vi "Create local tables from Server DB.vi"(6 "loadStatus Refnum":refnum<vi>, 8 "error in":errorcluster, 10 "Site":string="ICE1", 11 "tableNames":string[](array[string])) -> (0 "error out":errorcluster)   [LabVIEW 2015]
uses:
  <vilib>/addons/database/Auxilliary.llb/DB Tools DataTypes.ctl
  <vilib>/addons/database/Auxilliary.llb/DB Tools Cursor Type.ctl
  <vilib>/addons/database/Connection.llb/DB Tools Open Connec (Path).vi
  <vilib>/addons/database/Connection.llb/Conn Execute.vi
  <vilib>/addons/database/Recordset.llb/Rec Fetch Recordset Data (R).vi
  <vilib>/addons/database/Recordset.llb/Rec Destroy - Connection.vi
  <vilib>/addons/database/_DB Variant To Data/Database Variant To Data.xnode
  <vilib>/addons/database/NI_Database_API.lvlib
panel:
  out "column information":T2(array[cluster])
  out "columns":string[](array[string])
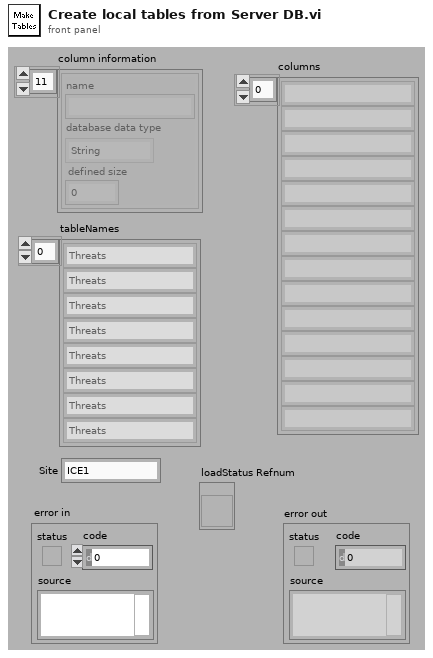
[diagram p1: front panel]
types:
  T1 = typedef "NI_Database_API.lvlib/DB Tools DataTypes.ctl" = enum16{"String", "Long (I32)", "Single (SGL)", "Double (DBL)", "Date/Time", "Binary"}
  T2 = cluster{"name":string, "database data type":T1, "defined size":i32}[]
  T3 = typedef "NI_Database_API.lvlib/DB Tools Cursor Type.ctl" = enum16{"forward-only", "keyset", "dynamic", "static"}
  T4 = typedef "NI_Database_API.lvlib/Conn ObjectReference.ctl" = refnum<k1>
  T5 = typedef "NI_Database_API.lvlib/Rec ObjectReference.ctl" = refnum<k1>
  T6 = cluster{"data":i32, "data":i32, "data":i32, "trimmed string":string, "trimmed string":string, "data":i32, "data":sgl, "data":i32, "data":i32, "data":i32, "trimmed string":string}
  T7 = cluster{"data":i32, "data":i32, "data":i32, "trimmed string":string, "data":i32, "data":i32, "trimmed string":string, "trimmed string":string, "trimmed string":string, "data":i32, "data":i32, "data":sgl, "data":i32, "data":i32, "trimmed string":string, "trimmed string":string}
  T8 = cluster{"data":i32, "trimmed string":string, "data":i32, "data":i32}
  T9 = cluster{"data":i32, "trimmed string":string, "data":i32, "trimmed string":string, "trimmed string":string, "trimmed string":string, "trimmed string":string, "data":sgl, "data":string, "trimmed string":string, "data":i32, "trimmed string":string, "trimmed string":string, "trimmed string":string}
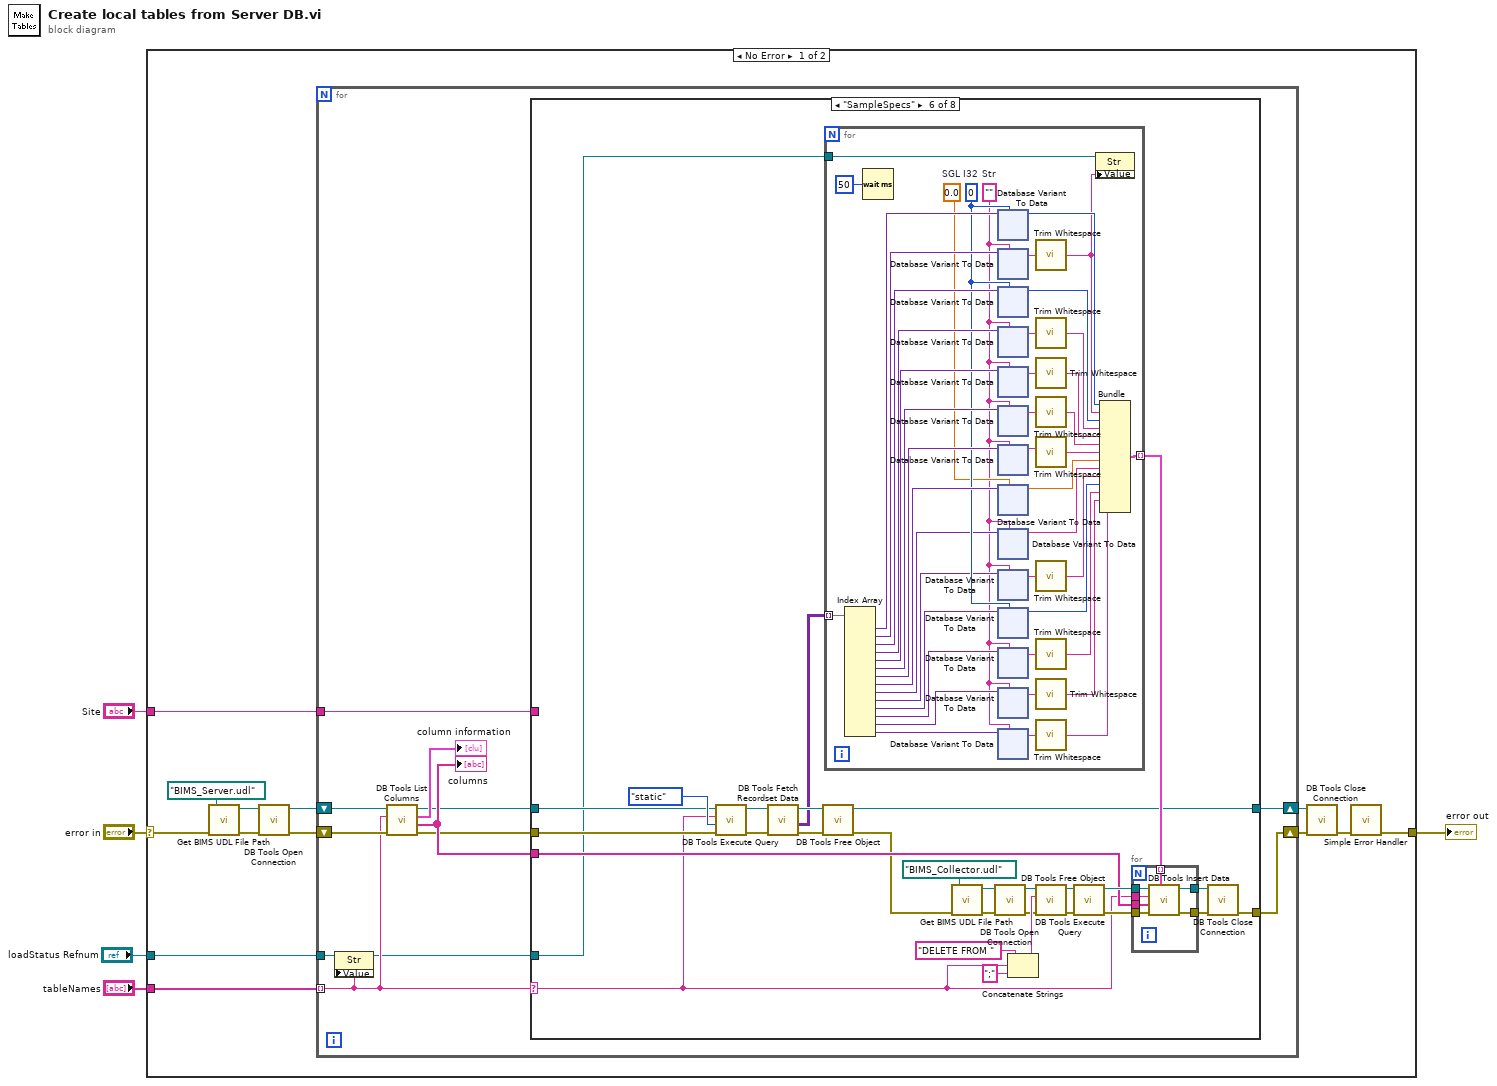
[diagram p0: block diagram]
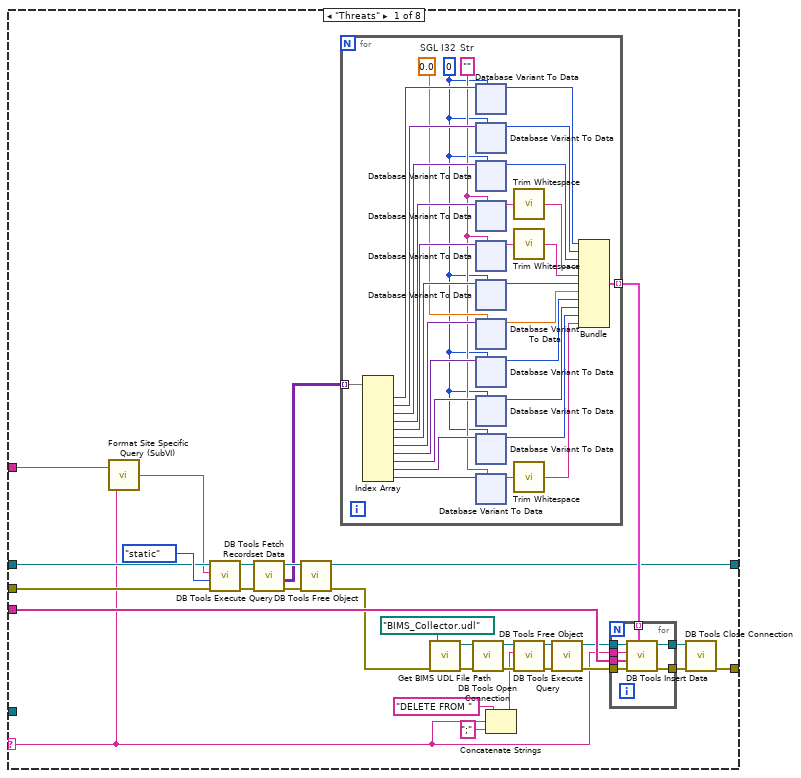
[diagram p2: hidden frame]
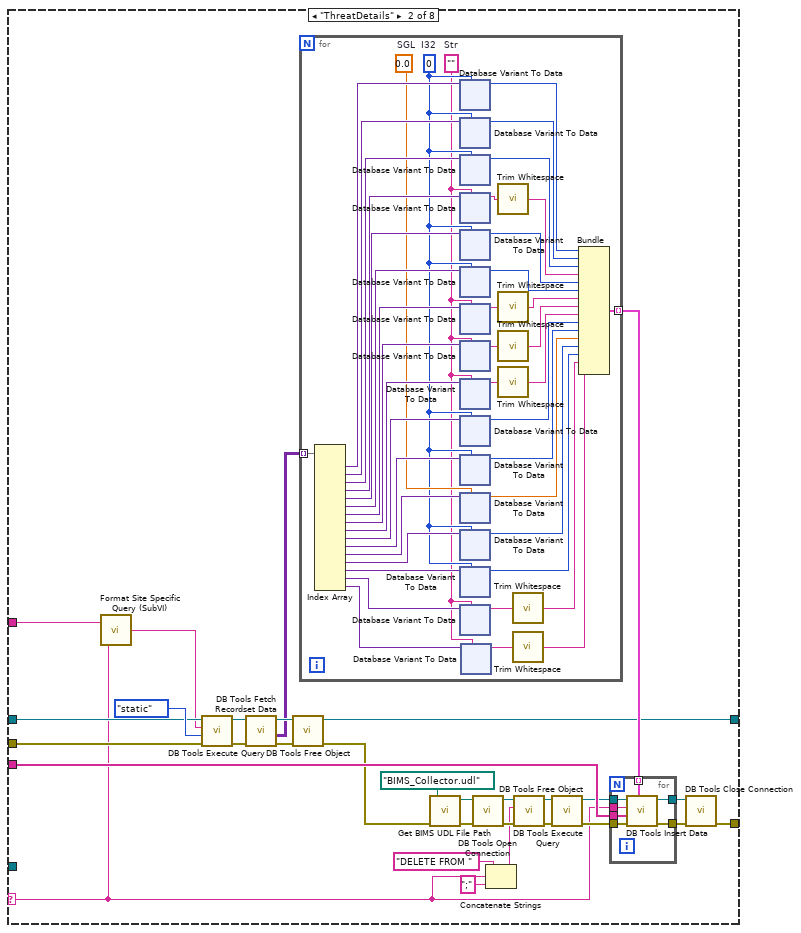
[diagram p3: hidden frame]
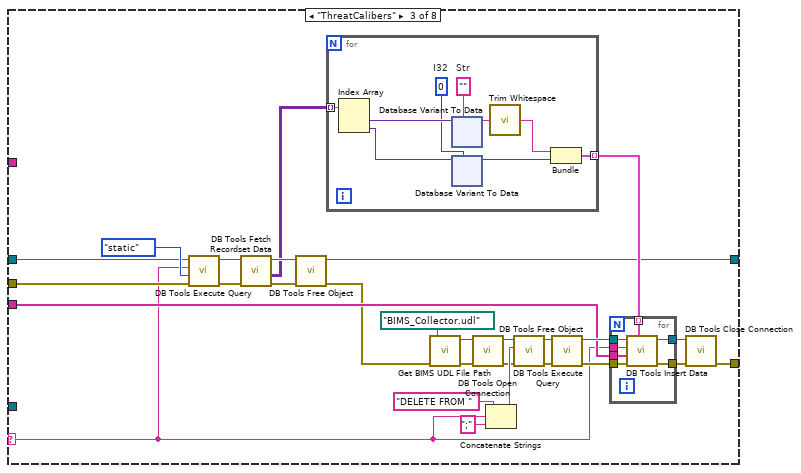
[diagram p4: hidden frame]
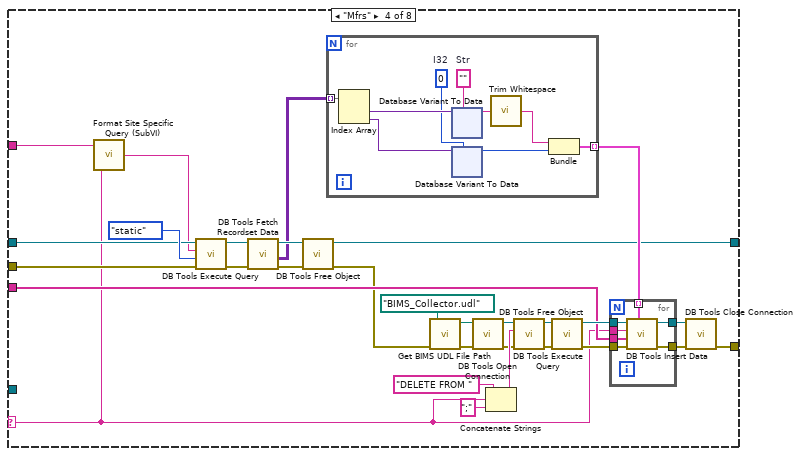
[diagram p5: hidden frame]
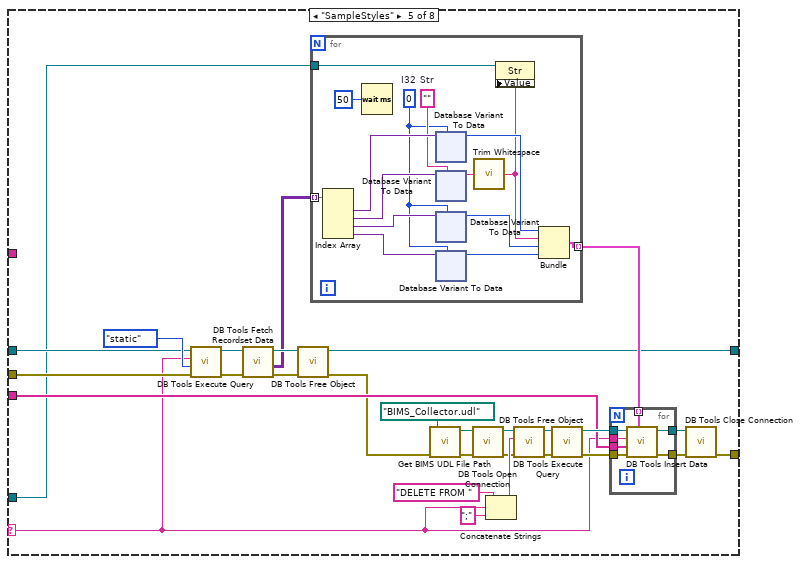
[diagram p6: hidden frame]
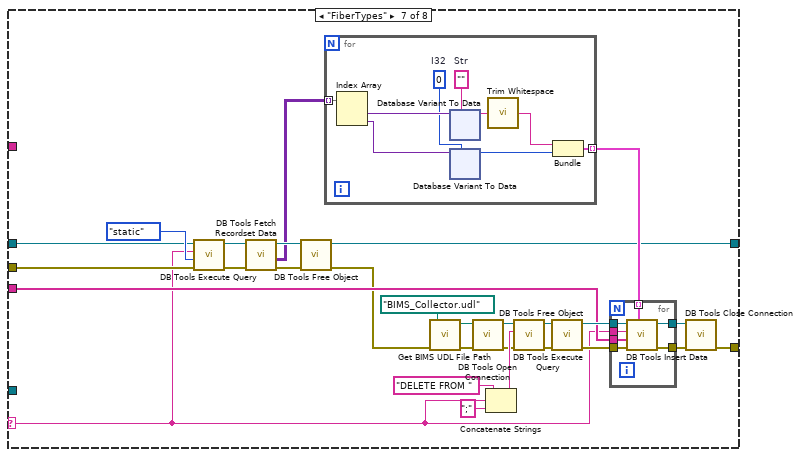
[diagram p7: hidden frame]
diagram:
  n1 = case shown="No Error" "error in" {
    selector: "error in" -> [w12 w2077]
    tunnel: [w16 w2077] -> w2
    tunnel: "tableNames" -> [w18 _]
    tunnel: "Site" -> [w17 _]
    tunnel: "loadStatus Refnum" -> [w6 _]
    frame No Error {
      n2 = call "Get BIMS UDL File Path.vi"("error in"=w12, "UDL file name"=path "BIMS_Server.udl") -> ("error out"=w15:errorcluster, "Full UDL file path"=w14:path)  [unwired: 4 out]
      n3 = call-poly <vilib>:"DB Tools Open Connection.vi"("error in (no error)"=w15, "connection information"=w14) -> ("error out"=w11:errorcluster, "connection reference"=w9:T4)  [unwired: 3 in, 3 out]
      n4 = for {
        tunnel: w18 -> [w20] mode=indexing
        shift-right: [w28] -> w8
        shift-left: w11 -> [w24]
        tunnel: w17 -> [w26]
        shift-right: [w23] -> w10
        shift-left: w9 -> [w22]
        tunnel: w6 -> [w21]
        n5 = property class="Str"(reference=w21, "Value"=w20) -> (reference out=w19:refnum<vi>)  [unwired: 1 in, 1 out]
        n6 = call <vilib>:"DB Tools List Columns.vi"("error in (no error)"=w24, "table"=w20, "connection reference"=w22) -> ("error out"=w27:errorcluster, "columns"=w29:string[], "column information"=→"column information":T2, "connection reference out"=w25:T4)  [unwired: 1 out]
        "columns" <- w29
        n7 = case shown="\"SampleSpecs\"" w20 {
          selector: w20 -> [w34 w453 w1046 w1154 w1265 w1440 w1971 _]
          tunnel: w27 -> [w39 w458 w1048 w1158 w1267 w1446 w1972 w2076]
          tunnel: w29 -> [w58 w477 w1055 w1165 w1274 w1454 w1981 _]
          tunnel: [w45 w464 w1054 w1164 w1273 w1453 w1980 w2076] -> w28
          tunnel: w25 -> [w38 w457 w1047 w1157 w1264 w1445 w1970 w2075]
          tunnel: w26 -> [w35 w454 _ w1155 _ _ _ _]
          tunnel: [w32 w450 w1043 w1151 w1262 w1442 w1967 w2075] -> w23
          tunnel: w19 -> [_ _ _ _ w1260 w1439 _ _]
          frame "Threats" {
            n8 = call "Format Site Specific Query (SubVI).vi"("Table"=w34, "Site"=w35) -> ("Query"=w36:string)
            n9 = call-poly <vilib>:"DB Tools Execute Query.vi"("error in (no error)"=w39, "cursor type"=DB_Tools_Cursor_Type."static", "SQL query"=w36, "connection reference"=w38) -> ("error out"=w43:errorcluster, "recordset reference"=w42:T5)  [unwired: 4 out]
            n10 = call-poly <vilib>:"DB Tools Fetch Recordset Data.vi"("error in (no error)"=w43, "recordset reference"=w42) -> ("error out"=w40:errorcluster, "recordset data"=w37:variant[][], "recordset reference out"=w41:T5)  [unwired: 3 out]
            n11 = call-poly <vilib>:"DB Tools Free Object.vi"("error in (no error)"=w40, "recordset reference"=w41) -> ("error out"=w31:errorcluster, "connection reference"=w32:T4)  [unwired: 8 out]
            n12 = for {
              tunnel: [w76] -> w55 mode=indexing
              tunnel: w37 -> [w97] mode=indexing
              w83 = sgl 0.0  # SGL
              w78 = ""  # Str
              w74 = 0  # I32
              n13 = Index Array(array=w97) -> (element #1=w96:variant, element #2=w95:variant, element #3=w92:variant, element #4=w91:variant, element #5=w90:variant, element #6=w89:variant, element #7=w88:variant, element #8=w87:variant, element #9=w82:variant, element #10=w80:variant, element #11=w77:variant)  [unwired: 11 in]
              n14 = xnode ("Database Variant To Data")("database variant"=w96, "type"=w74) -> ("data"=w75:i32)  [unwired: 1 in, 1 out]
              n15 = xnode "Database Variant To Data"("database variant"=w95, "type"=w74) -> ("data"=w94:i32)  [unwired: 1 in, 1 out]
              n16 = xnode "Database Variant To Data"("database variant"=w92, "type"=w74) -> ("data"=w93:i32)  [unwired: 1 in, 1 out]
              n17 = xnode "Database Variant To Data"("database variant"=w91, "type"=w78) -> ("data"=w73:string)  [unwired: 1 in, 1 out]
              n18 = xnode ("Database Variant To Data")("database variant"=w90, "type"=w78) -> ("data"=w71:string)  [unwired: 1 in, 1 out]
              n19 = xnode "Database Variant To Data"("database variant"=w89, "type"=w74) -> ("data"=w86:i32)  [unwired: 1 in, 1 out]
              n20 = xnode "Database Variant To Data"("database variant"=w88, "type"=w83) -> ("data"=w85:sgl)  [unwired: 1 in, 1 out]
              n21 = xnode "Database Variant To Data"("database variant"=w87, "type"=w74) -> ("data"=w84:i32)  [unwired: 1 in, 1 out]
              n22 = xnode "Database Variant To Data"("database variant"=w82, "type"=w74) -> ("data"=w81:i32)  [unwired: 1 in, 1 out]
              n23 = xnode "Database Variant To Data"("database variant"=w80, "type"=w74) -> ("data"=w79:i32)  [unwired: 1 in, 1 out]
              n24 = xnode "Database Variant To Data"("database variant"=w77, "type"=w78) -> ("data"=w69:string)  [unwired: 1 in, 1 out]
              n25 = call <vilib>:"Trim Whitespace.vi"("string"=w73) -> ("trimmed string"=w72:string)  [unwired: 1 in]
              n26 = call <vilib>:"Trim Whitespace.vi"("string"=w71) -> ("trimmed string"=w70:string)  [unwired: 1 in]
              n27 = call <vilib>:"Trim Whitespace.vi"("string"=w69) -> ("trimmed string"=w68:string)  [unwired: 1 in]
              n28 = Bundle("data"=w75, "data"=w94, "data"=w93, "trimmed string"=w72, "trimmed string"=w70, "data"=w86, "data"=w85, "data"=w84, "data"=w81, "data"=w79, "trimmed string"=w68) -> (w76:T6)  [unwired: 1 out]
            }
            n29 = call "Get BIMS UDL File Path.vi"("error in"=w31, "UDL file name"=path "BIMS_Collector.udl") -> ("error out"=w33:errorcluster, "Full UDL file path"=w60:path)  [unwired: 4 out]
            n30 = call-poly <vilib>:"DB Tools Open Connection.vi"("error in (no error)"=w33, "connection information"=w60) -> ("error out"=w54:errorcluster, "connection reference"=w51:T4)  [unwired: 3 in, 3 out]
            n31 = Concatenate Strings("DELETE FROM " ("SQL query"), w34, ";" ("string")) -> (w52:string)
            n32 = call-poly <vilib>:"DB Tools Execute Query.vi"("error in (no error)"=w54, "SQL query"=w52, "connection reference"=w51) -> ("error out"=w49:errorcluster, "recordset reference"=w47:T5)  [unwired: 1 in, 4 out]
            n33 = call-poly <vilib>:"DB Tools Free Object.vi"("error in (no error)"=w49, "recordset reference"=w47) -> ("error out"=w48:errorcluster, "connection reference"=w46:T4)  [unwired: 8 out]
            n34 = for {
              tunnel: [w67] -> w56
              tunnel: [w63] -> w57
              tunnel: w48 -> [w66]
              tunnel: w34 -> [w65]
              tunnel: w55 -> [w62] mode=indexing
              tunnel: w58 -> [w64]
              tunnel: w46 -> [w61]
              n35 = call <vilib>:"DB Tools Insert Data.vi"("data"=w62, "error in (no error)"=w66, "columns"=w64, "table"=w65, "connection reference"=w61) -> ("error out"=w63:errorcluster, "connection reference out"=w67:T4)  [unwired: 2 in, 3 out]
            }
            n36 = call <vilib>:"DB Tools Close Connection.vi"("error in (no error)"=w57, "connection reference"=w56) -> ("error out"=w45:errorcluster)  [unwired: 5 out]
          }
          frame "ThreatDetails" {
            n37 = call "Format Site Specific Query (SubVI).vi"("Table"=w453, "Site"=w454) -> ("Query"=w455:string)
            n38 = call-poly <vilib>:"DB Tools Execute Query.vi"("error in (no error)"=w458, "cursor type"=DB_Tools_Cursor_Type."static", "SQL query"=w455, "connection reference"=w457) -> ("error out"=w462:errorcluster, "recordset reference"=w461:T5)  [unwired: 4 out]
            n39 = call-poly <vilib>:"DB Tools Fetch Recordset Data.vi"("error in (no error)"=w462, "recordset reference"=w461) -> ("error out"=w459:errorcluster, "recordset data"=w456:variant[][], "recordset reference out"=w460:T5)  [unwired: 3 out]
            n40 = call-poly <vilib>:"DB Tools Free Object.vi"("error in (no error)"=w459, "recordset reference"=w460) -> ("error out"=w451:errorcluster, "connection reference"=w450:T4)  [unwired: 8 out]
            n41 = for {
              tunnel: [w513] -> w474 mode=indexing
              tunnel: w456 -> [w529] mode=indexing
              w500 = sgl 0.0  # SGL
              w489 = ""  # Str
              w496 = 0  # I32
              n42 = Index Array(array=w529) -> (element #1=w528:variant, element #2=w527:variant, element #3=w524:variant, element #4=w523:variant, element #5=w522:variant, element #6=w521:variant, element #7=w520:variant, element #8=w519:variant, element #9=w517:variant, element #10=w516:variant, element #11=w514:variant, element #12=w503:variant, element #13=w502:variant, element #14=w501:variant, element #15=w495:variant, element #16=w487:variant)  [unwired: 16 in]
              n43 = xnode ("Database Variant To Data")("database variant"=w528, "type"=w496) -> ("data"=w512:i32)  [unwired: 1 in, 1 out]
              n44 = xnode "Database Variant To Data"("database variant"=w527, "type"=w496) -> ("data"=w526:i32)  [unwired: 1 in, 1 out]
              n45 = xnode "Database Variant To Data"("database variant"=w524, "type"=w496) -> ("data"=w525:i32)  [unwired: 1 in, 1 out]
              n46 = xnode "Database Variant To Data"("database variant"=w523, "type"=w489) -> ("data"=w511:string)  [unwired: 1 in, 1 out]
              n47 = xnode ("Database Variant To Data")("database variant"=w522, "type"=w496) -> ("data"=w509:i32)  [unwired: 1 in, 1 out]
              n48 = xnode "Database Variant To Data"("database variant"=w521, "type"=w496) -> ("data"=w518:i32)  [unwired: 1 in, 1 out]
              n49 = xnode "Database Variant To Data"("database variant"=w520, "type"=w489) -> ("data"=w492:string)  [unwired: 1 in, 1 out]
              n50 = xnode "Database Variant To Data"("database variant"=w519, "type"=w489) -> ("data"=w508:string)  [unwired: 1 in, 1 out]
              n51 = xnode "Database Variant To Data"("database variant"=w517, "type"=w489) -> ("data"=w506:string)  [unwired: 1 in, 1 out]
              n52 = xnode "Database Variant To Data"("database variant"=w516, "type"=w496) -> ("data"=w515:i32)  [unwired: 1 in, 1 out]
              n53 = xnode "Database Variant To Data"("database variant"=w514, "type"=w496) -> ("data"=w504:i32)  [unwired: 1 in, 1 out]
              n54 = xnode "Database Variant To Data"("database variant"=w503, "type"=w500) -> ("data"=w499:sgl)  [unwired: 1 in, 1 out]
              n55 = xnode "Database Variant To Data"("database variant"=w502, "type"=w496) -> ("data"=w498:i32)  [unwired: 1 in, 1 out]
              n56 = xnode "Database Variant To Data"("database variant"=w501, "type"=w496) -> ("data"=w497:i32)  [unwired: 1 in, 1 out]
              n57 = xnode "Database Variant To Data"("database variant"=w495, "type"=w489) -> ("data"=w494:string)  [unwired: 1 in, 1 out]
              n58 = xnode "Database Variant To Data"("database variant"=w487, "type"=w489) -> ("data"=w490:string)  [unwired: 1 in, 1 out]
              n59 = call <vilib>:"Trim Whitespace.vi"("string"=w511) -> ("trimmed string"=w510:string)  [unwired: 1 in]
              n60 = call <vilib>:"Trim Whitespace.vi"("string"=w492) -> ("trimmed string"=w491:string)  [unwired: 1 in]
              n61 = call <vilib>:"Trim Whitespace.vi"("string"=w508) -> ("trimmed string"=w507:string)  [unwired: 1 in]
              n62 = call <vilib>:"Trim Whitespace.vi"("string"=w506) -> ("trimmed string"=w505:string)  [unwired: 1 in]
              n63 = call <vilib>:"Trim Whitespace.vi"("string"=w494) -> ("trimmed string"=w493:string)  [unwired: 1 in]
              n64 = call <vilib>:"Trim Whitespace.vi"("string"=w490) -> ("trimmed string"=w488:string)  [unwired: 1 in]
              n65 = Bundle("data"=w512, "data"=w526, "data"=w525, "trimmed string"=w510, "data"=w509, "data"=w518, "trimmed string"=w491, "trimmed string"=w507, "trimmed string"=w505, "data"=w515, "data"=w504, "data"=w499, "data"=w498, "data"=w497, "trimmed string"=w493, "trimmed string"=w488) -> (w513:T7)  [unwired: 1 out]
            }
            n66 = call "Get BIMS UDL File Path.vi"("error in"=w451, "UDL file name"=path "BIMS_Collector.udl") -> ("error out"=w452:errorcluster, "Full UDL file path"=w479:path)  [unwired: 4 out]
            n67 = call-poly <vilib>:"DB Tools Open Connection.vi"("error in (no error)"=w452, "connection information"=w479) -> ("error out"=w473:errorcluster, "connection reference"=w470:T4)  [unwired: 3 in, 3 out]
            n68 = Concatenate Strings("DELETE FROM " ("SQL query"), w453, ";" ("string")) -> (w471:string)
            n69 = call-poly <vilib>:"DB Tools Execute Query.vi"("error in (no error)"=w473, "SQL query"=w471, "connection reference"=w470) -> ("error out"=w468:errorcluster, "recordset reference"=w466:T5)  [unwired: 1 in, 4 out]
            n70 = call-poly <vilib>:"DB Tools Free Object.vi"("error in (no error)"=w468, "recordset reference"=w466) -> ("error out"=w467:errorcluster, "connection reference"=w465:T4)  [unwired: 8 out]
            n71 = for {
              tunnel: [w486] -> w475
              tunnel: [w482] -> w476
              tunnel: w467 -> [w485]
              tunnel: w453 -> [w484]
              tunnel: w474 -> [w481] mode=indexing
              tunnel: w477 -> [w483]
              tunnel: w465 -> [w480]
              n72 = call <vilib>:"DB Tools Insert Data.vi"("data"=w481, "error in (no error)"=w485, "columns"=w483, "table"=w484, "connection reference"=w480) -> ("error out"=w482:errorcluster, "connection reference out"=w486:T4)  [unwired: 2 in, 3 out]
            }
            n73 = call <vilib>:"DB Tools Close Connection.vi"("error in (no error)"=w476, "connection reference"=w475) -> ("error out"=w464:errorcluster)  [unwired: 5 out]
          }
          frame "ThreatCalibers" {
            n74 = call-poly <vilib>:"DB Tools Execute Query.vi"("error in (no error)"=w1048, "cursor type"=DB_Tools_Cursor_Type."static", "SQL query"=w1046, "connection reference"=w1047) -> ("error out"=w1051:errorcluster, "recordset reference"=w1050:T5)  [unwired: 4 out]
            n75 = call-poly <vilib>:"DB Tools Fetch Recordset Data.vi"("error in (no error)"=w1051, "recordset reference"=w1050) -> ("error out"=w1052:errorcluster, "recordset data"=w1045:variant[][], "recordset reference out"=w1049:T5)  [unwired: 3 out]
            n76 = call-poly <vilib>:"DB Tools Free Object.vi"("error in (no error)"=w1052, "recordset reference"=w1049) -> ("error out"=w1042:errorcluster, "connection reference"=w1043:T4)  [unwired: 8 out]
            n77 = for {
              tunnel: [w1081] -> w1060 mode=indexing
              tunnel: w1045 -> [w1085] mode=indexing
              w1077 = ""  # Str
              w1078 = 0  # I32
              n78 = Index Array(array=w1085) -> (element #1=w1084:variant, element #2=w1083:variant)  [unwired: 2 in]
              n79 = xnode ("Database Variant To Data")("database variant"=w1084, "type"=w1077) -> ("data"=w1080:string)  [unwired: 1 in, 1 out]
              n80 = xnode "Database Variant To Data"("database variant"=w1083, "type"=w1078) -> ("data"=w1082:i32)  [unwired: 1 in, 1 out]
              n81 = call <vilib>:"Trim Whitespace.vi"("string"=w1080) -> ("trimmed string"=w1079:string)  [unwired: 1 in]
              n82 = Bundle("trimmed string"=w1079, "data"=w1082) -> (w1081:cluster{"trimmed string":string, "data":i32})  [unwired: 1 out]
            }
            n83 = call "Get BIMS UDL File Path.vi"("error in"=w1042, "UDL file name"=path "BIMS_Collector.udl") -> ("error out"=w1044:errorcluster, "Full UDL file path"=w1056:path)  [unwired: 4 out]
            n84 = call-poly <vilib>:"DB Tools Open Connection.vi"("error in (no error)"=w1044, "connection information"=w1056) -> ("error out"=w1061:errorcluster, "connection reference"=w1064:T4)  [unwired: 3 in, 3 out]
            n85 = Concatenate Strings("DELETE FROM " ("SQL query"), w1046, ";" ("string")) -> (w1063:string)
            n86 = call-poly <vilib>:"DB Tools Execute Query.vi"("error in (no error)"=w1061, "SQL query"=w1063, "connection reference"=w1064) -> ("error out"=w1066:errorcluster, "recordset reference"=w1068:T5)  [unwired: 1 in, 4 out]
            n87 = call-poly <vilib>:"DB Tools Free Object.vi"("error in (no error)"=w1066, "recordset reference"=w1068) -> ("error out"=w1067:errorcluster, "connection reference"=w1069:T4)  [unwired: 8 out]
            n88 = for {
              tunnel: [w1076] -> w1059
              tunnel: [w1072] -> w1058
              tunnel: w1067 -> [w1075]
              tunnel: w1046 -> [w1074]
              tunnel: w1060 -> [w1071] mode=indexing
              tunnel: w1055 -> [w1073]
              tunnel: w1069 -> [w1070]
              n89 = call <vilib>:"DB Tools Insert Data.vi"("data"=w1071, "error in (no error)"=w1075, "columns"=w1073, "table"=w1074, "connection reference"=w1070) -> ("error out"=w1072:errorcluster, "connection reference out"=w1076:T4)  [unwired: 2 in, 3 out]
            }
            n90 = call <vilib>:"DB Tools Close Connection.vi"("error in (no error)"=w1058, "connection reference"=w1059) -> ("error out"=w1054:errorcluster)  [unwired: 5 out]
          }
          frame "Mfrs" {
            n91 = call "Format Site Specific Query (SubVI).vi"("Table"=w1154, "Site"=w1155) -> ("Query"=w1153:string)
            n92 = call-poly <vilib>:"DB Tools Execute Query.vi"("error in (no error)"=w1158, "cursor type"=DB_Tools_Cursor_Type."static", "SQL query"=w1153, "connection reference"=w1157) -> ("error out"=w1161:errorcluster, "recordset reference"=w1160:T5)  [unwired: 4 out]
            n93 = call-poly <vilib>:"DB Tools Fetch Recordset Data.vi"("error in (no error)"=w1161, "recordset reference"=w1160) -> ("error out"=w1162:errorcluster, "recordset data"=w1156:variant[][], "recordset reference out"=w1159:T5)  [unwired: 3 out]
            n94 = call-poly <vilib>:"DB Tools Free Object.vi"("error in (no error)"=w1162, "recordset reference"=w1159) -> ("error out"=w1150:errorcluster, "connection reference"=w1151:T4)  [unwired: 8 out]
            n95 = for {
              tunnel: [w1193] -> w1170 mode=indexing
              tunnel: w1156 -> [w1195] mode=indexing
              w1190 = ""  # Str
              w1189 = 0  # I32
              n96 = Index Array(array=w1195) -> (element #1=w1191:variant, element #2=w1194:variant)  [unwired: 2 in]
              n97 = xnode "Database Variant To Data"("database variant"=w1191, "type"=w1190) -> ("data"=w1188:string)  [unwired: 1 in, 1 out]
              n98 = xnode ("Database Variant To Data")("database variant"=w1194, "type"=w1189) -> ("data"=w1187:i32)  [unwired: 1 in, 1 out]
              n99 = call <vilib>:"Trim Whitespace.vi"("string"=w1188) -> ("trimmed string"=w1192:string)  [unwired: 1 in]
              n100 = Bundle("trimmed string"=w1192, "data"=w1187) -> (w1193:cluster{"trimmed string":string, "data":i32})  [unwired: 1 out]
            }
            n101 = call "Get BIMS UDL File Path.vi"("error in"=w1150, "UDL file name"=path "BIMS_Collector.udl") -> ("error out"=w1152:errorcluster, "Full UDL file path"=w1166:path)  [unwired: 4 out]
            n102 = call-poly <vilib>:"DB Tools Open Connection.vi"("error in (no error)"=w1152, "connection information"=w1166) -> ("error out"=w1171:errorcluster, "connection reference"=w1174:T4)  [unwired: 3 in, 3 out]
            n103 = Concatenate Strings("DELETE FROM " ("SQL query"), w1154, ";" ("string")) -> (w1173:string)
            n104 = call-poly <vilib>:"DB Tools Execute Query.vi"("error in (no error)"=w1171, "SQL query"=w1173, "connection reference"=w1174) -> ("error out"=w1176:errorcluster, "recordset reference"=w1178:T5)  [unwired: 1 in, 4 out]
            n105 = call-poly <vilib>:"DB Tools Free Object.vi"("error in (no error)"=w1176, "recordset reference"=w1178) -> ("error out"=w1177:errorcluster, "connection reference"=w1179:T4)  [unwired: 8 out]
            n106 = for {
              tunnel: [w1186] -> w1169
              tunnel: [w1182] -> w1168
              tunnel: w1177 -> [w1185]
              tunnel: w1154 -> [w1184]
              tunnel: w1170 -> [w1181] mode=indexing
              tunnel: w1165 -> [w1183]
              tunnel: w1179 -> [w1180]
              n107 = call <vilib>:"DB Tools Insert Data.vi"("data"=w1181, "error in (no error)"=w1185, "columns"=w1183, "table"=w1184, "connection reference"=w1180) -> ("error out"=w1182:errorcluster, "connection reference out"=w1186:T4)  [unwired: 2 in, 3 out]
            }
            n108 = call <vilib>:"DB Tools Close Connection.vi"("error in (no error)"=w1168, "connection reference"=w1169) -> ("error out"=w1164:errorcluster)  [unwired: 5 out]
          }
          frame "SampleStyles" {
            n109 = call-poly <vilib>:"DB Tools Execute Query.vi"("error in (no error)"=w1267, "cursor type"=DB_Tools_Cursor_Type."static", "SQL query"=w1265, "connection reference"=w1264) -> ("error out"=w1270:errorcluster, "recordset reference"=w1269:T5)  [unwired: 4 out]
            n110 = call-poly <vilib>:"DB Tools Fetch Recordset Data.vi"("error in (no error)"=w1270, "recordset reference"=w1269) -> ("error out"=w1271:errorcluster, "recordset data"=w1266:variant[][], "recordset reference out"=w1268:T5)  [unwired: 3 out]
            n111 = call-poly <vilib>:"DB Tools Free Object.vi"("error in (no error)"=w1271, "recordset reference"=w1268) -> ("error out"=w1261:errorcluster, "connection reference"=w1262:T4)  [unwired: 8 out]
            n112 = for {
              tunnel: [w1306] -> w1279 mode=indexing
              tunnel: w1266 -> [w1310] mode=indexing
              tunnel: w1260 -> [w1298]
              w1303 = ""  # Str
              w1302 = 0  # I32
              n113 = Index Array(array=w1310) -> (element #1=w1304:variant, element #2=w1305:variant, element #3=w1309:variant, element #4=w1308:variant)  [unwired: 4 in]
              n114 = Wait (ms)(milliseconds to wait=u32 50) -> ()  [unwired: 1 out]
              n115 = xnode ("Database Variant To Data")("database variant"=w1304, "type"=w1302) -> ("data"=w1300:i32)  [unwired: 1 in, 1 out]
              n116 = xnode "Database Variant To Data"("database variant"=w1305, "type"=w1303) -> ("data"=w1301:string)  [unwired: 1 in, 1 out]
              n117 = xnode ("Database Variant To Data")("database variant"=w1309, "type"=w1302) -> ("data"=w1299:i32)  [unwired: 1 in, 1 out]
              n118 = xnode "Database Variant To Data"("database variant"=w1308, "type"=w1302) -> ("data"=w1307:i32)  [unwired: 1 in, 1 out]
              n119 = call <vilib>:"Trim Whitespace.vi"("string"=w1301) -> ("trimmed string"=w1297:string)  [unwired: 1 in]
              n120 = property class="Str"(reference=w1298, "Value"=w1297) -> ()  [unwired: 1 in, 2 out]
              n121 = Bundle("data"=w1300, "trimmed string"=w1297, "data"=w1299, "data"=w1307) -> (w1306:T8)  [unwired: 1 out]
            }
            n122 = call "Get BIMS UDL File Path.vi"("error in"=w1261, "UDL file name"=path "BIMS_Collector.udl") -> ("error out"=w1263:errorcluster, "Full UDL file path"=w1275:path)  [unwired: 4 out]
            n123 = call-poly <vilib>:"DB Tools Open Connection.vi"("error in (no error)"=w1263, "connection information"=w1275) -> ("error out"=w1280:errorcluster, "connection reference"=w1283:T4)  [unwired: 3 in, 3 out]
            n124 = Concatenate Strings("DELETE FROM " ("SQL query"), w1265, ";" ("string")) -> (w1282:string)
            n125 = call-poly <vilib>:"DB Tools Execute Query.vi"("error in (no error)"=w1280, "SQL query"=w1282, "connection reference"=w1283) -> ("error out"=w1285:errorcluster, "recordset reference"=w1287:T5)  [unwired: 1 in, 4 out]
            n126 = call-poly <vilib>:"DB Tools Free Object.vi"("error in (no error)"=w1285, "recordset reference"=w1287) -> ("error out"=w1286:errorcluster, "connection reference"=w1288:T4)  [unwired: 8 out]
            n127 = for {
              tunnel: [w1295] -> w1278
              tunnel: [w1291] -> w1277
              tunnel: w1286 -> [w1294]
              tunnel: w1265 -> [w1293]
              tunnel: w1279 -> [w1290] mode=indexing
              tunnel: w1274 -> [w1292]
              tunnel: w1288 -> [w1289]
              n128 = call <vilib>:"DB Tools Insert Data.vi"("data"=w1290, "error in (no error)"=w1294, "columns"=w1292, "table"=w1293, "connection reference"=w1289) -> ("error out"=w1291:errorcluster, "connection reference out"=w1295:T4)  [unwired: 2 in, 3 out]
            }
            n129 = call <vilib>:"DB Tools Close Connection.vi"("error in (no error)"=w1277, "connection reference"=w1278) -> ("error out"=w1273:errorcluster)  [unwired: 5 out]
          }
          frame "SampleSpecs" {
            n130 = call-poly <vilib>:"DB Tools Execute Query.vi"("error in (no error)"=w1446, "cursor type"=DB_Tools_Cursor_Type."static", "SQL query"=w1440, "connection reference"=w1445) -> ("error out"=w1449:errorcluster, "recordset reference"=w1448:T5)  [unwired: 4 out]
            n131 = call-poly <vilib>:"DB Tools Fetch Recordset Data.vi"("error in (no error)"=w1449, "recordset reference"=w1448) -> ("error out"=w1450:errorcluster, "recordset data"=w1444:variant[][], "recordset reference out"=w1447:T5)  [unwired: 3 out]
            n132 = call-poly <vilib>:"DB Tools Free Object.vi"("error in (no error)"=w1450, "recordset reference"=w1447) -> ("error out"=w1441:errorcluster, "connection reference"=w1442:T4)  [unwired: 8 out]
            n133 = for {
              tunnel: [w1499] -> w1452 mode=indexing
              tunnel: w1444 -> [w1511] mode=indexing
              tunnel: w1439 -> [w1468]
              w1475 = sgl 0.0  # SGL
              w1472 = ""  # Str
              w1497 = 0  # I32
              n134 = Index Array(array=w1511) -> (element #1=w1510:variant, element #2=w1509:variant, element #3=w1507:variant, element #4=w1506:variant, element #5=w1505:variant, element #6=w1504:variant, element #7=w1503:variant, element #8=w1502:variant, element #9=w1476:variant, element #10=w1477:variant, element #11=w1478:variant, element #12=w1479:variant, element #13=w1480:variant, element #14=w1473:variant)  [unwired: 14 in]
              n135 = Wait (ms)(milliseconds to wait=u32 50) -> ()  [unwired: 1 out]
              n136 = xnode ("Database Variant To Data")("database variant"=w1510, "type"=w1497) -> ("data"=w1498:i32)  [unwired: 1 in, 1 out]
              n137 = xnode "Database Variant To Data"("database variant"=w1509, "type"=w1472) -> ("data"=w1490:string)  [unwired: 1 in, 1 out]
              n138 = xnode "Database Variant To Data"("database variant"=w1507, "type"=w1497) -> ("data"=w1508:i32)  [unwired: 1 in, 1 out]
              n139 = xnode "Database Variant To Data"("database variant"=w1506, "type"=w1472) -> ("data"=w1496:string)  [unwired: 1 in, 1 out]
              n140 = xnode ("Database Variant To Data")("database variant"=w1505, "type"=w1472) -> ("data"=w1494:string)  [unwired: 1 in, 1 out]
              n141 = xnode "Database Variant To Data"("database variant"=w1504, "type"=w1472) -> ("data"=w1485:string)  [unwired: 1 in, 1 out]
              n142 = xnode "Database Variant To Data"("database variant"=w1503, "type"=w1472) -> ("data"=w1487:string)  [unwired: 1 in, 1 out]
              n143 = xnode "Database Variant To Data"("database variant"=w1502, "type"=w1475) -> ("data"=w1501:sgl)  [unwired: 1 in, 1 out]
              n144 = xnode "Database Variant To Data"("database variant"=w1476, "type"=w1472) -> ("data"=w1481:string)  [unwired: 1 in, 1 out]
              n145 = xnode "Database Variant To Data"("database variant"=w1477, "type"=w1472) -> ("data"=w1489:string)  [unwired: 1 in, 1 out]
              n146 = xnode "Database Variant To Data"("database variant"=w1478, "type"=w1497) -> ("data"=w1500:i32)  [unwired: 1 in, 1 out]
              n147 = xnode "Database Variant To Data"("database variant"=w1479, "type"=w1472) -> ("data"=w1492:string)  [unwired: 1 in, 1 out]
              n148 = xnode "Database Variant To Data"("database variant"=w1480, "type"=w1472) -> ("data"=w1483:string)  [unwired: 1 in, 1 out]
              n149 = xnode "Database Variant To Data"("database variant"=w1473, "type"=w1472) -> ("data"=w1474:string)  [unwired: 1 in, 1 out]
              n150 = call <vilib>:"Trim Whitespace.vi"("string"=w1490) -> ("trimmed string"=w1469:string)  [unwired: 1 in]
              n151 = call <vilib>:"Trim Whitespace.vi"("string"=w1496) -> ("trimmed string"=w1495:string)  [unwired: 1 in]
              n152 = call <vilib>:"Trim Whitespace.vi"("string"=w1494) -> ("trimmed string"=w1493:string)  [unwired: 1 in]
              n153 = call <vilib>:"Trim Whitespace.vi"("string"=w1485) -> ("trimmed string"=w1484:string)  [unwired: 1 in]
              n154 = call <vilib>:"Trim Whitespace.vi"("string"=w1487) -> ("trimmed string"=w1486:string)  [unwired: 1 in]
              n155 = call <vilib>:"Trim Whitespace.vi"("string"=w1489) -> ("trimmed string"=w1488:string)  [unwired: 1 in]
              n156 = call <vilib>:"Trim Whitespace.vi"("string"=w1492) -> ("trimmed string"=w1491:string)  [unwired: 1 in]
              n157 = call <vilib>:"Trim Whitespace.vi"("string"=w1483) -> ("trimmed string"=w1482:string)  [unwired: 1 in]
              n158 = call <vilib>:"Trim Whitespace.vi"("string"=w1474) -> ("trimmed string"=w1471:string)  [unwired: 1 in]
              n159 = property class="Str"(reference=w1468, "Value"=w1469) -> ()  [unwired: 1 in, 2 out]
              n160 = Bundle("data"=w1498, "trimmed string"=w1469, "data"=w1508, "trimmed string"=w1495, "trimmed string"=w1493, "trimmed string"=w1484, "trimmed string"=w1486, "data"=w1501, "data"=w1481, "trimmed string"=w1488, "data"=w1500, "trimmed string"=w1491, "trimmed string"=w1482, "trimmed string"=w1471) -> (w1499:T9)  [unwired: 1 out]
            }
            n161 = call "Get BIMS UDL File Path.vi"("error in"=w1441, "UDL file name"=path "BIMS_Collector.udl") -> ("error out"=w1443:errorcluster, "Full UDL file path"=w1455:path)  [unwired: 4 out]
            n162 = call-poly <vilib>:"DB Tools Open Connection.vi"("error in (no error)"=w1443, "connection information"=w1455) -> ("error out"=w1459:errorcluster, "connection reference"=w1462:T4)  [unwired: 3 in, 3 out]
            n163 = Concatenate Strings("DELETE FROM " ("SQL query"), w1440, ";" ("string")) -> (w1461:string)
            n164 = call-poly <vilib>:"DB Tools Execute Query.vi"("error in (no error)"=w1459, "SQL query"=w1461, "connection reference"=w1462) -> ("error out"=w1464:errorcluster, "recordset reference"=w1466:T5)  [unwired: 1 in, 4 out]
            n165 = call-poly <vilib>:"DB Tools Free Object.vi"("error in (no error)"=w1464, "recordset reference"=w1466) -> ("error out"=w1465:errorcluster, "connection reference"=w1467:T4)  [unwired: 8 out]
            n166 = for {
              tunnel: [w1966] -> w1458
              tunnel: [w1962] -> w1457
              tunnel: w1465 -> [w1965]
              tunnel: w1440 -> [w1964]
              tunnel: w1452 -> [w1961] mode=indexing
              tunnel: w1454 -> [w1963]
              tunnel: w1467 -> [w1960]
              n167 = call <vilib>:"DB Tools Insert Data.vi"("data"=w1961, "error in (no error)"=w1965, "columns"=w1963, "table"=w1964, "connection reference"=w1960) -> ("error out"=w1962:errorcluster, "connection reference out"=w1966:T4)  [unwired: 2 in, 3 out]
            }
            n168 = call <vilib>:"DB Tools Close Connection.vi"("error in (no error)"=w1457, "connection reference"=w1458) -> ("error out"=w1453:errorcluster)  [unwired: 5 out]
          }
          frame "FiberTypes" {
            n169 = call-poly <vilib>:"DB Tools Execute Query.vi"("error in (no error)"=w1972, "cursor type"=DB_Tools_Cursor_Type."static", "SQL query"=w1971, "connection reference"=w1970) -> ("error out"=w1977:errorcluster, "recordset reference"=w1976:T5)  [unwired: 4 out]
            n170 = call-poly <vilib>:"DB Tools Fetch Recordset Data.vi"("error in (no error)"=w1977, "recordset reference"=w1976) -> ("error out"=w1974:errorcluster, "recordset data"=w1973:variant[][], "recordset reference out"=w1975:T5)  [unwired: 3 out]
            n171 = call-poly <vilib>:"DB Tools Free Object.vi"("error in (no error)"=w1974, "recordset reference"=w1975) -> ("error out"=w1968:errorcluster, "connection reference"=w1967:T4)  [unwired: 8 out]
            n172 = for {
              tunnel: [w1999] -> w1979 mode=indexing
              tunnel: w1973 -> [w2003] mode=indexing
              w1995 = ""  # Str
              w1996 = 0  # I32
              n173 = Index Array(array=w2003) -> (element #1=w2002:variant, element #2=w2001:variant)  [unwired: 2 in]
              n174 = xnode ("Database Variant To Data")("database variant"=w2002, "type"=w1995) -> ("data"=w1998:string)  [unwired: 1 in, 1 out]
              n175 = xnode "Database Variant To Data"("database variant"=w2001, "type"=w1996) -> ("data"=w2000:i32)  [unwired: 1 in, 1 out]
              n176 = call <vilib>:"Trim Whitespace.vi"("string"=w1998) -> ("trimmed string"=w1997:string)  [unwired: 1 in]
              n177 = Bundle("trimmed string"=w1997, "data"=w2000) -> (w1999:cluster{"trimmed string":string, "data":i32})  [unwired: 1 out]
            }
            n178 = call "Get BIMS UDL File Path.vi"("error in"=w1968, "UDL file name"=path "BIMS_Collector.udl") -> ("error out"=w1969:errorcluster, "Full UDL file path"=w1982:path)  [unwired: 4 out]
            n179 = call-poly <vilib>:"DB Tools Open Connection.vi"("error in (no error)"=w1969, "connection information"=w1982) -> ("error out"=w1986:errorcluster, "connection reference"=w1989:T4)  [unwired: 3 in, 3 out]
            n180 = Concatenate Strings("DELETE FROM " ("SQL query"), w1971, ";" ("string")) -> (w1988:string)
            n181 = call-poly <vilib>:"DB Tools Execute Query.vi"("error in (no error)"=w1986, "SQL query"=w1988, "connection reference"=w1989) -> ("error out"=w1991:errorcluster, "recordset reference"=w1993:T5)  [unwired: 1 in, 4 out]
            n182 = call-poly <vilib>:"DB Tools Free Object.vi"("error in (no error)"=w1991, "recordset reference"=w1993) -> ("error out"=w1992:errorcluster, "connection reference"=w1994:T4)  [unwired: 8 out]
            n183 = for {
              tunnel: [w2074] -> w1985
              tunnel: [w2070] -> w1984
              tunnel: w1992 -> [w2073]
              tunnel: w1971 -> [w2072]
              tunnel: w1979 -> [w2069] mode=indexing
              tunnel: w1981 -> [w2071]
              tunnel: w1994 -> [w2068]
              n184 = call <vilib>:"DB Tools Insert Data.vi"("data"=w2069, "error in (no error)"=w2073, "columns"=w2071, "table"=w2072, "connection reference"=w2068) -> ("error out"=w2070:errorcluster, "connection reference out"=w2074:T4)  [unwired: 2 in, 3 out]
            }
            n185 = call <vilib>:"DB Tools Close Connection.vi"("error in (no error)"=w1984, "connection reference"=w1985) -> ("error out"=w1980:errorcluster)  [unwired: 5 out]
          }
          frame "Information", Default {
            # "The following case has a structure determined for \n  the Threats table in the BIMS server.\n\n  The data retieved from the table is site specific."
          }
        }
      }
      n186 = call <vilib>:"DB Tools Close Connection.vi"("error in (no error)"=w8, "connection reference"=w10) -> ("error out"=w7:errorcluster)  [unwired: 5 out]
      n187 = call <vilib>:"Simple Error Handler.vi"("error in (no error)"=w7) -> ("error out"=w16:errorcluster)  [unwired: 1 in, 7 out]
    }
    frame Error {
    }
  }
  "error out" <- w2
